vi "Delete Files From Memory.vi"(7 "MSUS":string, 8 "error in (no error)":errorcluster, 9 "File Name":string, 10 "File Type (0: Non Volatile User Files)":i32(ring) items=["Non Volatile User Files", "Binary Files", "Bit Files", "Arbitrary Waveform Digital Modulation Files", "FIR Files", "FSK Files", "IQ Files", "List Files", "Arbitrary Waveform Multicarrier Digital Modulation Files", "Arbitrary Waveform Multitone Files", "Pulse Train Files", "Sequence Files", "Burst Shape Files", "State Files", "User Flatness Files", "Select File", "Non Volatile Arbitrary Waveform Files", "Volatile Arbitrary Waveform Files", "Select File with MSUS"], 11 "VISA resource name":refnum<visa-resource-name>) -> (0 "error out":errorcluster, 3 "VISA resource name out":refnum<visa-resource-name>)   [LabVIEW 2018, in "Agilent PSG MXG Series.lvlib"]
doc: "Deletes files from memory. \n\n<B>Note:</B>\nThis VI is valid on N5171B, N5172B, N5173B, N5181B, N5182B, N5183B, N5161A, N5162A, N5181A, N5182A, N5183A."
uses:
  Agilent PSG MXG Series.lvlib
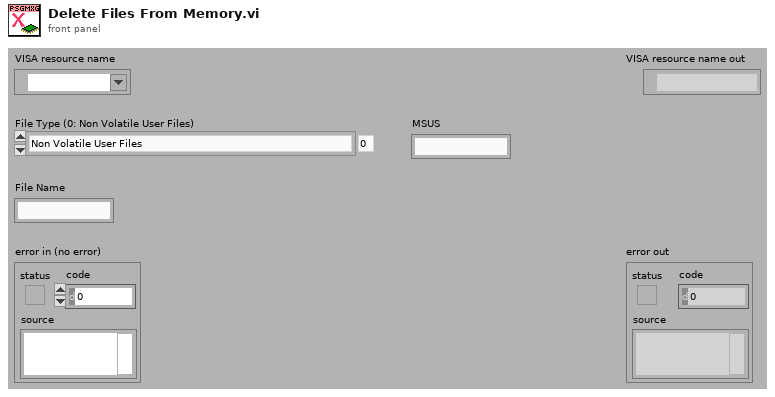
[diagram p1: front panel]
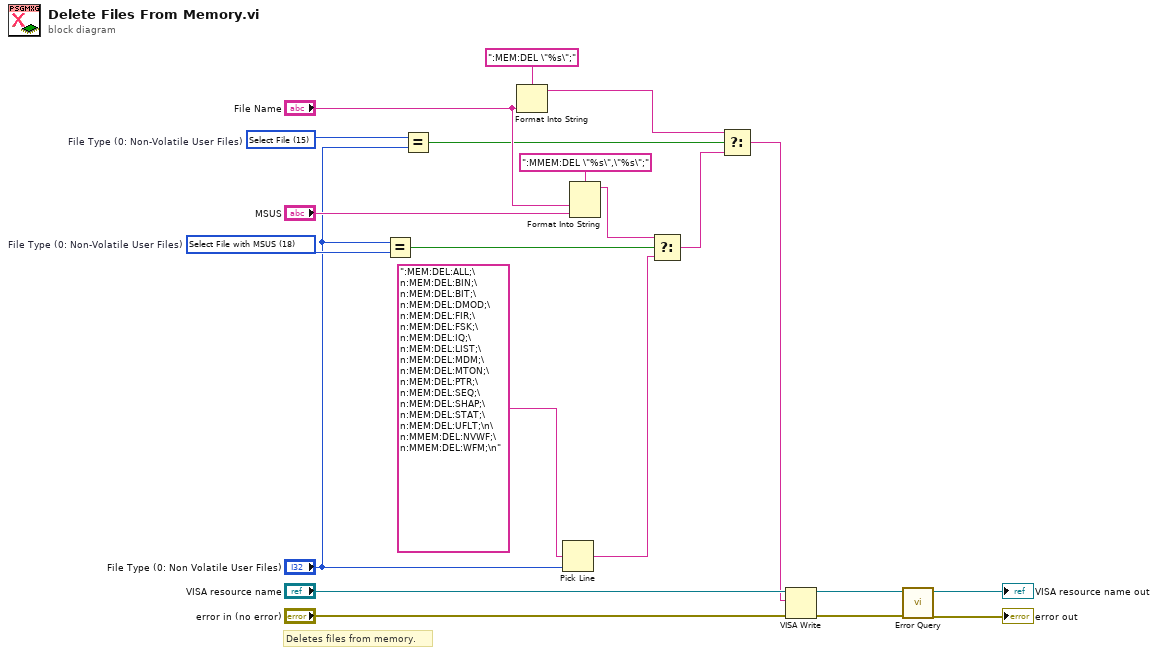
[diagram p0: block diagram]
diagram:
  w10 = 18 items=["Non-Volatile User Files", "Binary Files", "Bit Files", "Arbitrary Waveform Digital Modulation Files", "FIR Files", "FSK Files", "IQ Files", "List Files", "Arbitrary Waveform Multicarrier Digital Modulation Files", "Arbitrary Waveform Multitone Files", "Pulse Train Files", "Sequenc Files", "Burst Shape Files", "State Files", "User-Flatness Files", "Select File", "Non-Volatile Arbitrary Waveform Files", "Volatile Arbitrary Waveform Files", "Select File with MSUS"]  # File Type (0: Non-Volatile User Files)
  w5 = 15 items=["Non-Volatile User Files", "Binary Files", "Bit Files", "Arbitrary Waveform Digital Modulation Files", "FIR Files", "FSK Files", "IQ Files", "List Files", "Arbitrary Waveform Multicarrier Digital Modulation Files", "Arbitrary Waveform Multitone Files", "Pulse Train Files", "Sequenc Files", "Burst Shape Files", "State Files", "User-Flatness Files", "Select File", "Non-Volatile Arbitrary Waveform Files", "Volatile Arbitrary Waveform Files", "Select File with MSUS"]  # File Type (0: Non-Volatile User Files)
  # "Deletes files from memory."
  n1 = Equal?(x="File Type (0: Non Volatile User Files)", y=w10) -> (x = y?=w7:bool)
  n2 = Equal?(x=w5, y="File Type (0: Non Volatile User Files)") -> (x = y?=w9:bool)
  n3 = Format Into String(format string=":MEM:DEL \"%s\";", "File Name") -> (resulting string=w8:string)  [unwired: 2 in, 1 out]
  n4 = Pick Line(multi-line string=":MEM:DEL:ALL;\n:MEM:DEL:BIN;\n:MEM:DEL:BIT;\n:MEM:DEL:DMOD;\n:MEM:DEL:FIR;\n:MEM:DEL:FSK;\n:MEM:DEL:IQ;\n:MEM:DEL:LIST;\n:MEM:DEL:MDM;\n:MEM:DEL:MTON;\n:MEM:DEL:PTR;\n:MEM:DEL:SEQ;\n:MEM:DEL:SHAP;\n:MEM:DEL:STAT;\n:MEM:DEL:UFLT;\n\n:MMEM:DEL:NVWF;\n:MMEM:DEL:WFM;\n", line index="File Type (0: Non Volatile User Files)") -> (output string=w3:string)  [unwired: 1 in]
  n5 = Format Into String(format string=":MMEM:DEL \"%s\",\"%s\";", "File Name", "MSUS") -> (resulting string=w4:string)  [unwired: 2 in, 1 out]
  n6 = Select(t=w4, s=w7, f=w3) -> (s? t:f=w2:string)
  n7 = Select(t=w8, s=w9, f=w2) -> (s? t:f=w1:string)
  n8 = VISA Write(VISA resource name="VISA resource name", write buffer=w1, error in (no error)="error in (no error)") -> (VISA resource name out=w15:refnum<visa-resource-name>, error out=w14:errorcluster)  [unwired: 1 out]
  n9 = call "Error Query.vi"("error in (no error)"=w14, "VISA resource name"=w15) -> ("error out"=→"error out":errorcluster, "VISA resource name out"=→"VISA resource name out":refnum<visa-resource-name>)  [unwired: 6 in, 2 out]
